vi "Get Stylesheet.vi"(8 "error in":errorcluster, 11 "SpreadsheetDoc in":refnum<k24>) -> (0 "error out":errorcluster, 2 "Stylesheet":refnum<k24>, 3 "SpreadsheetDoc out":refnum<k24>)   [LabVIEW 2021, in "Open Xml.lvlib"]
uses:
  Open Xml.lvlib
  D:/git/Open-Xml-LabVIEW/dll/DocumentFormat.OpenXml.dll
  dll/DocumentFormat.OpenXml.dll
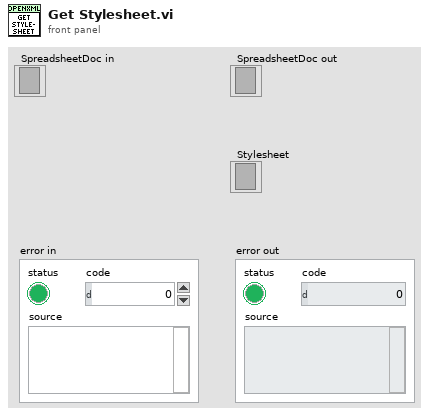
[diagram p1: front panel]
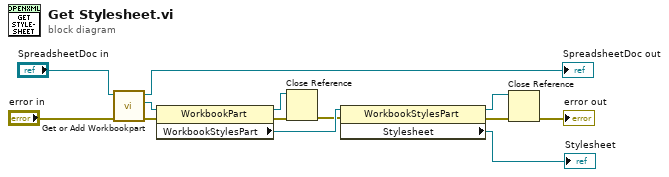
[diagram p0: block diagram]
diagram:
  n1 = call "Get or Add Workbookpart.vi"("error in"="error in", "SpreadsheetDocument"="SpreadsheetDoc in") -> ("error out"=w8:errorcluster, "WorkbookPart"=w10:refnum<k24>, "SpreadsheetDocument out"=→"SpreadsheetDoc out":refnum<k24>)  [unwired: 7 in]
  n2 = property class="WorkbookPart"(reference=w10, error in=w8) -> (reference out=w11:refnum<k24>, error out=w2:errorcluster, "WorkbookStylesPart"=w7:refnum<k24>)
  n3 = Close Reference(reference=w11, error in (no error)=w2) -> (error out=w1:errorcluster)
  n4 = property class="WorkbookStylesPart"(reference=w7, error in=w1) -> (reference out=w3:refnum<k24>, error out=w6:errorcluster, "Stylesheet"=→"Stylesheet":refnum<k24>)
  n5 = Close Reference(reference=w3, error in (no error)=w6) -> (error out=→"error out":errorcluster)
